vi "LoadDeviceList.vi"(6 "Error In":errorcluster, 9 "GAMRYCOMLib.IGamryDeviceList In":refnum<k7>) -> (0 "Error Out":errorcluster, 1 "EnumSections":variant, 2 "EnumLabels":variant, 3 "GAMRYCOMLib.IGamryDeviceList Out":refnum<k7>)   [LabVIEW 2016]
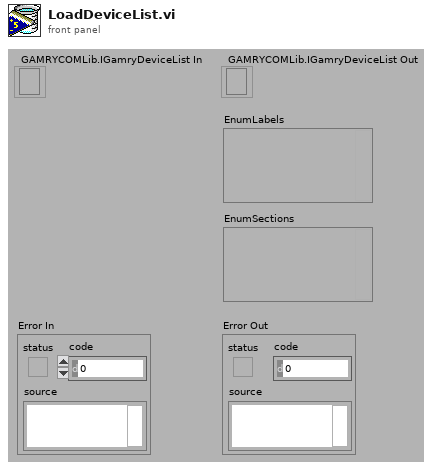
[diagram p1: front panel]
types:
  T1 = cluster{"status":bool, "code":u32, "source":string}
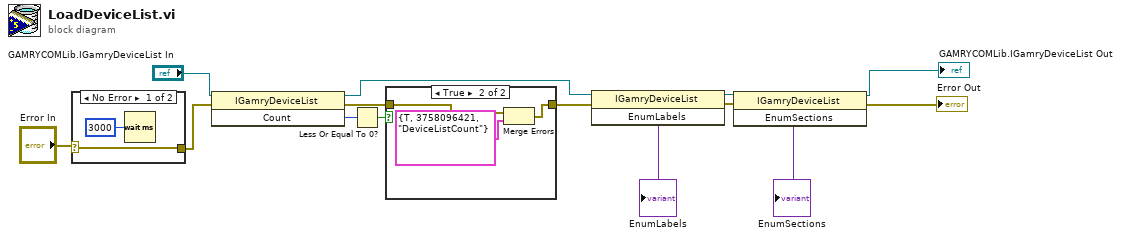
[diagram p0: block diagram]
diagram:
  n1 = case shown="No Error" "Error In" {
    selector: "Error In" -> [w15 w17]
    tunnel: [w15 w17] -> w12
    frame No Error {
      n2 = Wait (ms)(milliseconds to wait=u32 3000) -> ()  [unwired: 1 out]
    }
    frame Error {
    }
  }
  n3 = invoke class="IGamryDeviceList" method="Count"(reference="GAMRYCOMLib.IGamryDeviceList In", error in=w12) -> (reference out=w7:refnum<k7>, error out=w9:errorcluster, "Count"=w10:i32)  [unwired: 1 in]
  n4 = Less Or Equal To 0?(x=w10) -> (x <= 0?=w11:bool)
  n5 = case shown="True" w11 {
    tunnel: [w18 w21] -> w8
    tunnel: w9 -> [w18 w20]
    frame False {
    }
    frame True {
      n6 = Merge Errors(w20, T1 {"status"=TRUE, "code"=3758096421, "source"="DeviceListCount"} ("error out")) -> (w21:errorcluster)
    }
  }
  n7 = invoke class="IGamryDeviceList" method="EnumLabels"(reference=w7, error in=w8) -> (reference out=w6:refnum<k7>, error out=w5:errorcluster, "EnumLabels"=→"EnumLabels":variant)  [unwired: 1 in]
  n8 = invoke class="IGamryDeviceList" method="EnumSections"(reference=w6, error in=w5) -> (reference out=→"GAMRYCOMLib.IGamryDeviceList Out":refnum<k7>, error out=→"Error Out":errorcluster, "EnumSections"=→"EnumSections":variant)  [unwired: 1 in]
